vi "_Main_ByRuns_V2.0_3el_5el.vi"() -> ()   [LabVIEW 2017]
uses:
  <vilib>/Instr/_visa.llb/VISA Configure Serial Port (Instr).vi
panel:
  in  "5electrodes":bool=TRUE
  in  "WaveForm":i32(listbox)
  in  "Auto\nturn OFF":bool
  in  "Content":i32(listbox)
  out "LastTrigTimer, s":dbl
  in  "Graph every, cycle":dbl=10.0 min=1.0 max=100.0
  in  "SendPeriod, ms":dbl=100.0 min=10.0 max=10000.0
  out "RunsNeed":i32
  out "DAC1volt, V":dbl
  out "Time LOG":cluster{dbl[], dbl[]}(graph)
  out "LED2":bool
  out "LED1":bool
  out "TrigTimer, s":dbl
  out "Bytes at Port":u32
  out "RecTry":i32
  out "OutVoltage, V":dbl
  out "Field, kV/cm":dbl
  out "VoltageRes, V":dbl
  out "PlotPoints":cluster{"Time":dbl[], "Voltage":dbl[]}(graph)={"Time"=[0.0, 0.00037111111108161925, 0.000510833333311085, 0.0006505555555405509, 0.0007766666666915019, 0.0009172222221968695, 0.0010569444444263353, 0.0011958333333152243, 0.0013350000000274223], "Voltage"=[5.89, 5.89, 5.89, 5.89, 5.89, 5.89, 5.89, 5.89, 5.89]}
  out "VoltageBelow, V":dbl
  in  "Exposition, s":dbl=3.0
  out "Knob":u32
  out "Current, mA":dbl format="%#_4g"
  out "Channel 4, V":dbl format="%#_5g"
  out "Channel 3, V":dbl format="%#_5g"
  out "Channel 2, V":dbl format="%#_5g"
  out "Channel 1, V":dbl format="%#_5g"
  in  "Stop Button":bool
  in  "Start Button":bool
  in  "film H, nm":dbl=50.0
  out "VoltageArray, V":dbl[](array[numeric])
  out "Shutter Red":bool
  out "Shutter Green":bool
  in  "Frames In Run":u32=180
  out "Global Frame Done":u32
  out "Now is Run #":u32
  out "Frame In Run Done":u32
  in  "Step, V":dbl=1.0 min=0.01 max=50.0
  in  "Amplitude, V":dbl=1.0 min=0.1 max=50.0
  in  "LOG file":path
  in  "COM port":refnum<visa-resource-name>
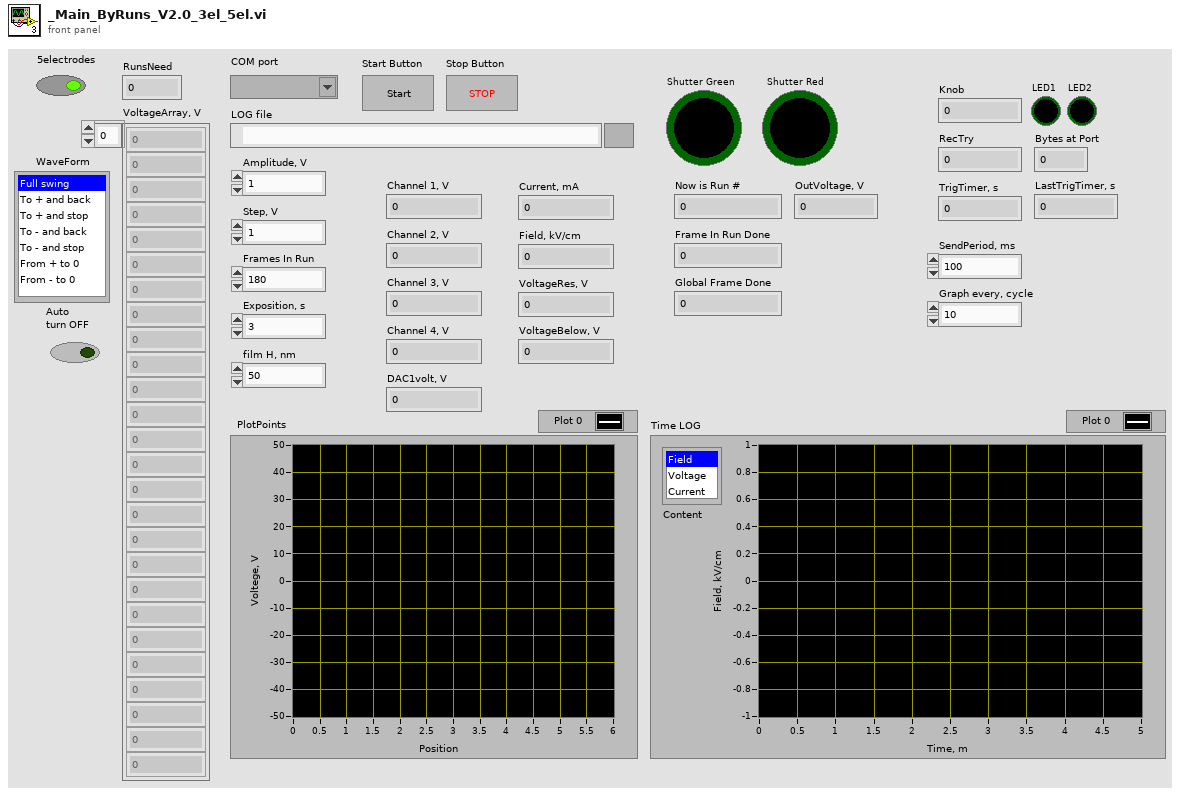
[diagram p1: front panel]
types:
  T1 = cluster{i32, i32, u32, "TrigState":bool, "TrigTimer, s":dbl, "CurrentError":bool}
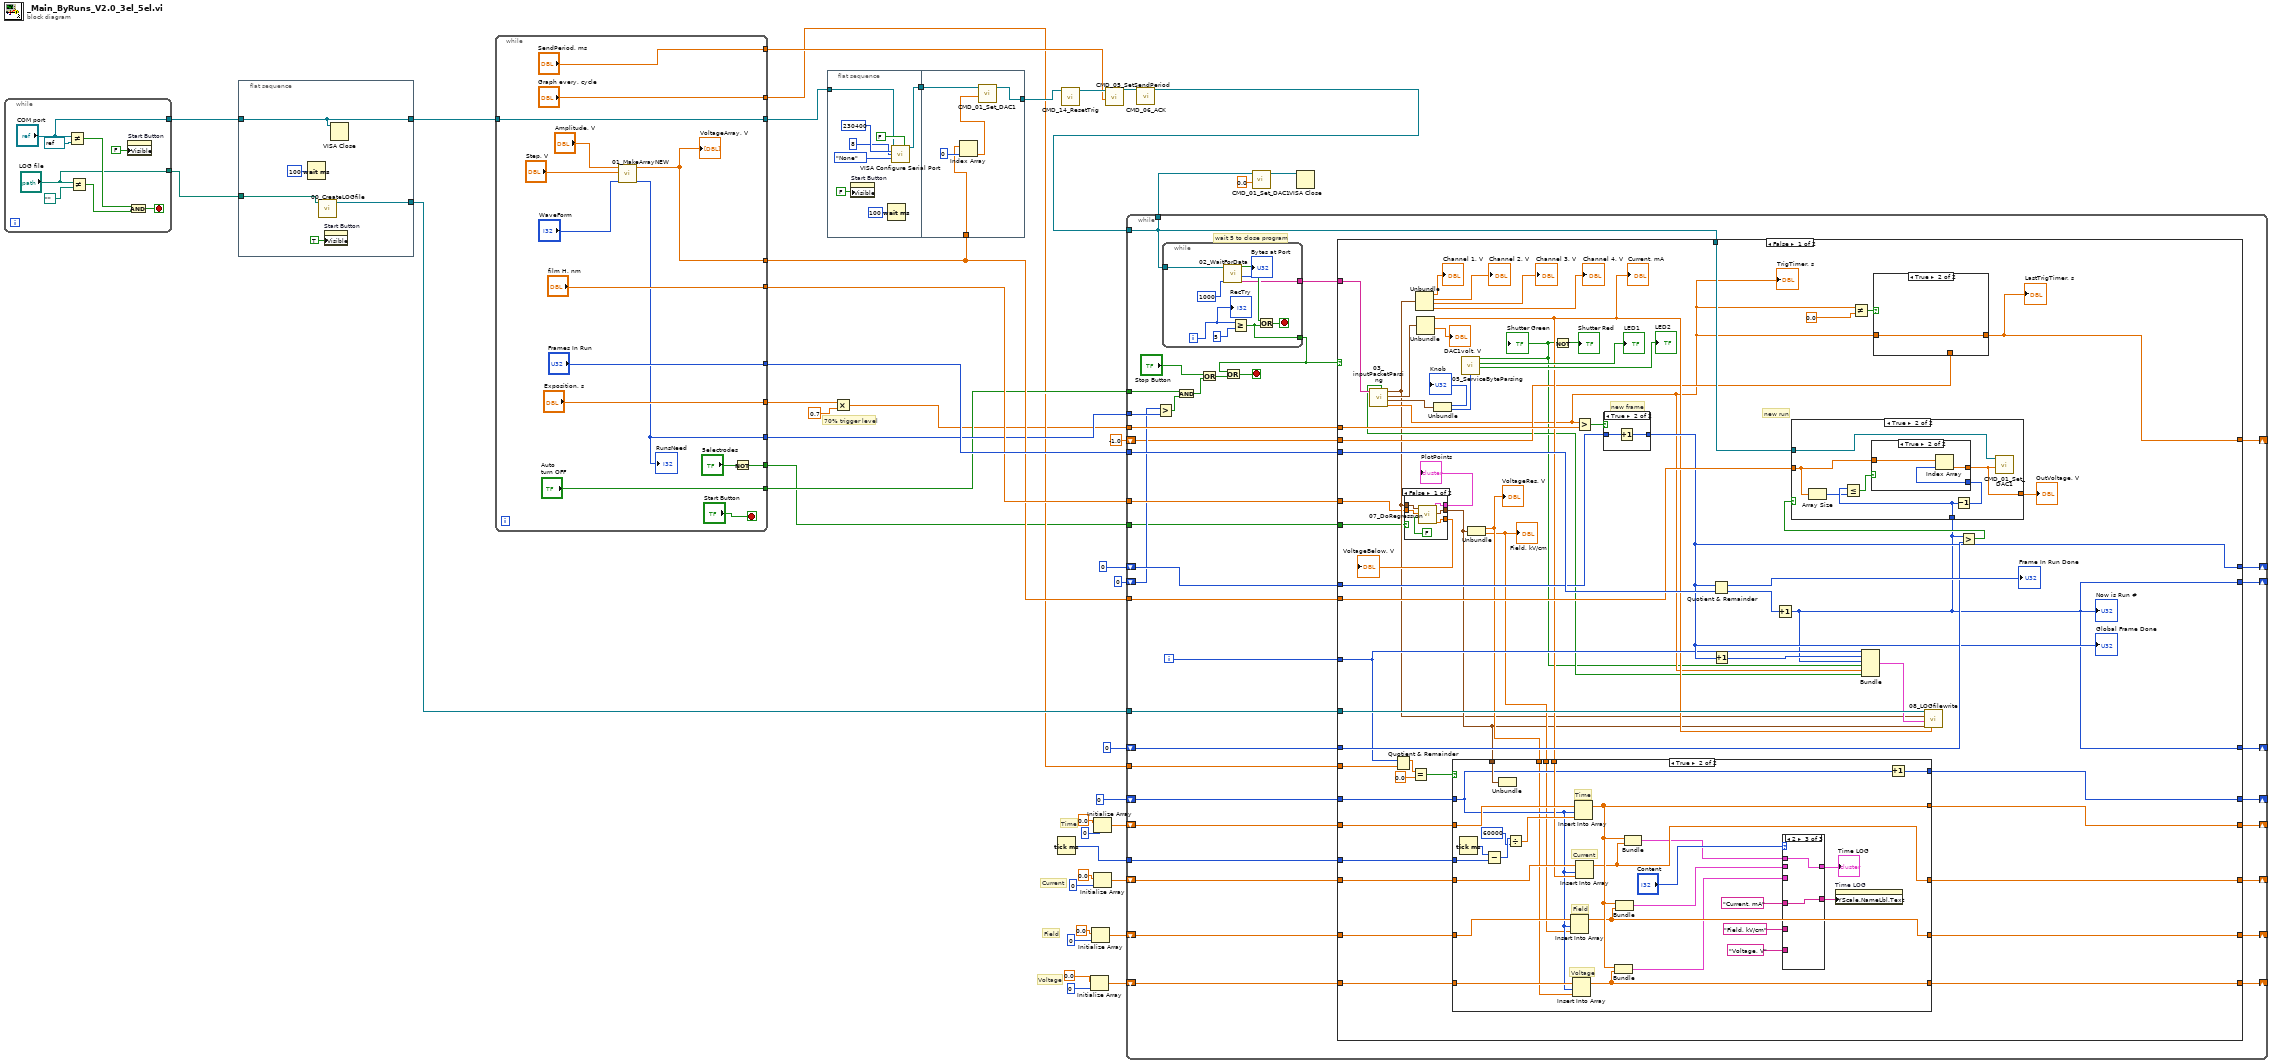
[diagram p0: block diagram]
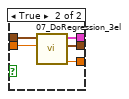
[diagram p2: hidden frame]
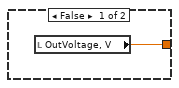
[diagram p7: hidden frame]
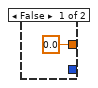
[diagram p8: hidden frame]
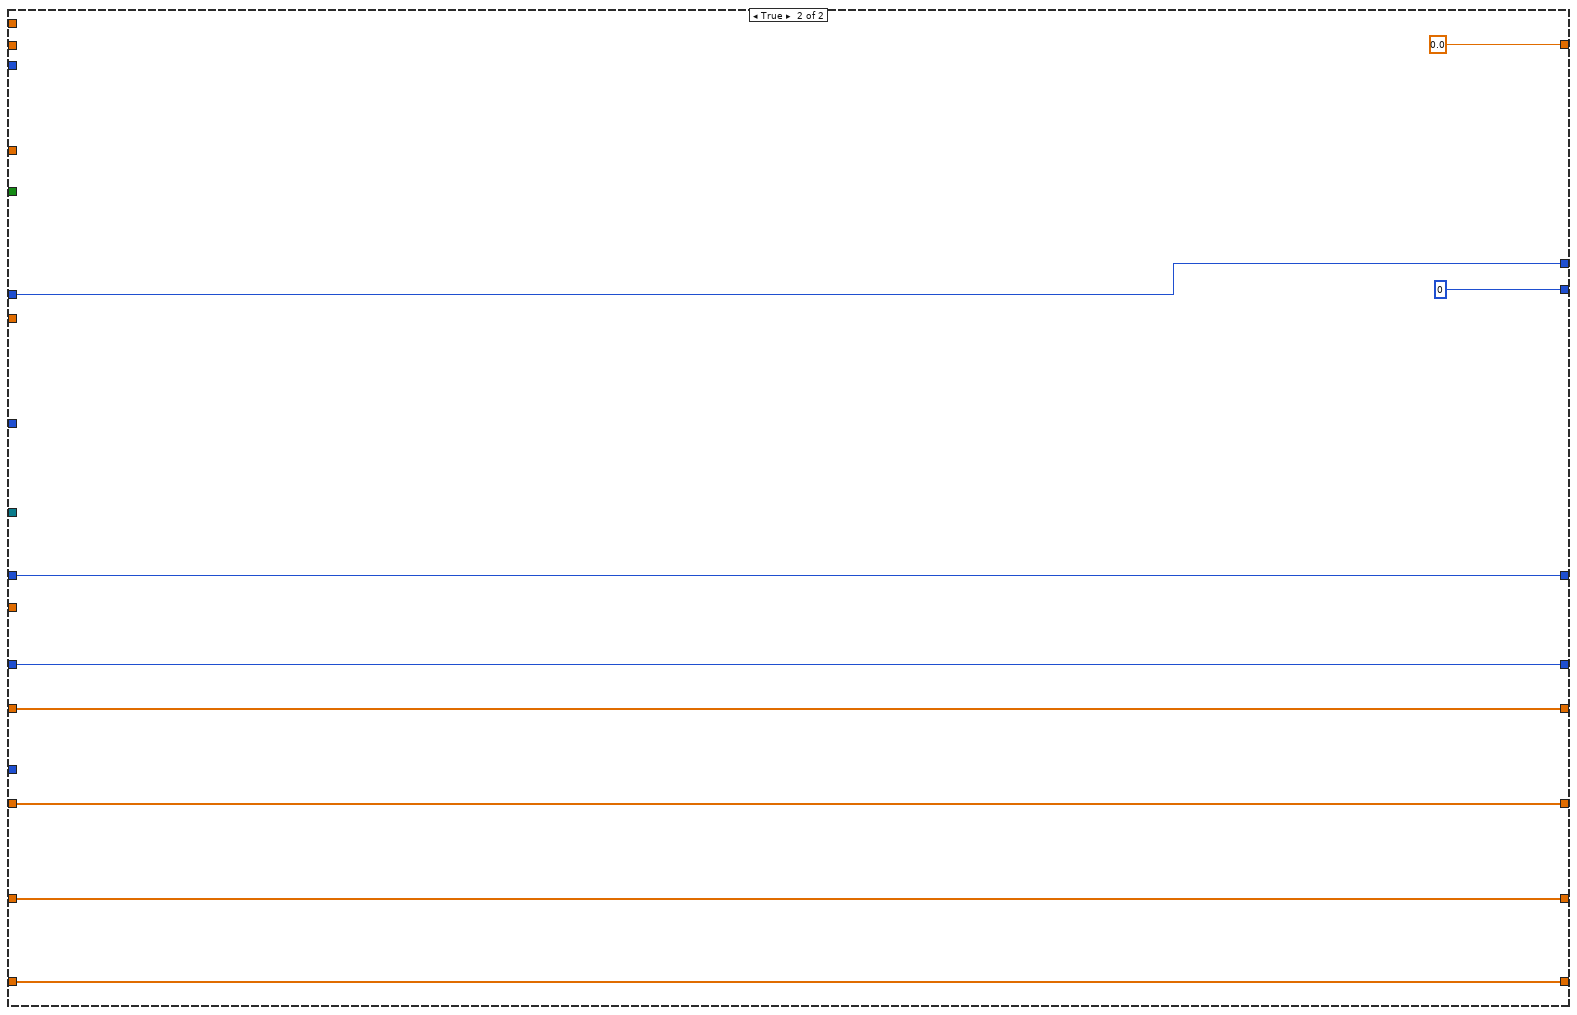
[diagram p10: hidden frame]
diagram:
  # "70% trigger level"
  # "Voltage"
  # "Field"
  # "Time"
  # "Current"
  n1 = while {
    tunnel: ["COM port"] -> w4
    tunnel: ["LOG file"] -> w3
    stop <- w48 stop-if-true
    n2 = Not Equal?(x="COM port", y=refnum<visa-resource-name> refnum ("COM port")) -> (x != y?=w45:bool)
    n3 = Not Equal?(x="LOG file", y=path "" ("LOG file")) -> (x != y?=w46:bool)
    n4 = property on="Start Button" class="Bool"("Visible"=FALSE) -> ()  [unwired: 2 in, 2 out]
    n5 = And(x=w45, y=w46) -> (x .and. y?=w48:bool)
  }
  n6 = flat-sequence {
    tunnel: [w55] -> w39
    tunnel: w4 -> [w51]
    tunnel: w3 -> [w52]
    tunnel: [w51] -> w2
    frame #0 {
      n7 = Wait (ms)(milliseconds to wait=u32 100) -> ()  [unwired: 1 out]
      n8 = call "00_CreateLOGfile.vi"("LOG file"=w52) -> ("refnum out"=w55:refnum<file>)  [unwired: 10 in]
      n9 = property on="Start Button" class="Bool"("Visible"=TRUE) -> ()  [unwired: 2 in, 2 out]
      n10 = VISA Close(VISA resource name=w51) -> ()  [unwired: 1 in, 1 out]
    }
  }
  n11 = while {
    tunnel: w2 -> [w62]
    tunnel: [w62] -> w42
    tunnel: [w59] -> w28
    tunnel: ["film H, nm"] -> w40
    tunnel: ["Frames In Run"] -> w41
    tunnel: ["Exposition, s"] -> w13
    tunnel: [w58] -> w19
    tunnel: ["Auto\nturn OFF"] -> w17
    tunnel: ["SendPeriod, ms"] -> w16
    tunnel: ["Graph every, cycle"] -> w15
    tunnel: [w57] -> w1
    stop <- "Start Button" stop-if-true
    n12 = call "01_MakeArrayNEW.vi"("Amp"="Amplitude, V", "Step"="Step, V", "WaveForm"="WaveForm") -> ("Array"=w59:dbl[], "ArraySize"=w58:i32)  [unwired: 6 in]
    "VoltageArray, V" <- w59
    "RunsNeed" <- w58
    n13 = Not(x="5electrodes") -> (.not. x?=w57:bool)
  }
  n14 = flat-sequence {
    tunnel: w42 -> [w74]
    tunnel: [w73] -> w29
    tunnel: [w81] -> w35
    tunnel: w29 -> [w80]
    tunnel: w28 -> [w79]
    frame #0 {
      n15 = property on="Start Button" class="Bool"("Visible"=FALSE) -> ()  [unwired: 2 in, 2 out]
      n16 = Wait (ms)(milliseconds to wait=u32 100) -> ()  [unwired: 1 out]
      n17 = call-poly "VISA Configure Serial Port"("VISA resource name"=w74, "Enable Termination\nChar (T)"=FALSE ("Enable Termination\nChar (T)"), "baud rate (9600)"=u32 230400, "data bits (8)"=u16 8, "parity (0:none)"=enum16{"None", "Odd", "Even", "Mark", "Space"}."None") -> ("VISA resource name out"=w73:refnum<visa-resource-name>)  [unwired: 9 in, 1 out]
    }
    frame #1 {
      n18 = Index Array(array=w79, index=0) -> (element=w83:dbl)
      n19 = call "CMD_01_Set_DAC1.vi"("Input, V"=w83, "VISA resource name"=w80) -> ("VISA resource name out"=w81:refnum<visa-resource-name>)  [unwired: 9 in]
    }
  }
  n20 = Multiply(x=w13, y=0.7) -> (x*y=w14:dbl)
  n21 = Tick Count (ms)() -> (millisecond timer value=w23:u32)
  n22 = call "CMD_14_ResetTrig.vi"("VISA resource name"=w35) -> ("VISA resource name out"=w32:refnum<visa-resource-name>)  [unwired: 10 in]
  n23 = Initialize Array(0.0 ("element"), 0 ("dimension size")) -> (w5:dbl[])
  n24 = Initialize Array(0.0 ("element"), 0 ("dimension size")) -> (w6:dbl[])
  n25 = Initialize Array(0.0 ("element"), 0 ("dimension size")) -> (w20:dbl[])
  n26 = Initialize Array(0.0 ("element"), 0 ("dimension size")) -> (w24:dbl[])
  n27 = call "CMD_05_SetSendPeriod.vi"("Period, ms"=w16, "VISA resource name"=w32) -> ("VISA resource name out"=w31:refnum<visa-resource-name>)  [unwired: 9 in]
  n28 = call "CMD_06_ACK.vi"("VISA resource name"=w31) -> ("VISA resource name out"=w30:refnum<visa-resource-name>)  [unwired: 10 in]
  n29 = while {
    tunnel: w30 -> [w107]
    tunnel: [w107] -> w36
    tunnel: w28 -> [w108]
    tunnel: w41 -> [w114]
    tunnel: w14 -> [w116]
    tunnel: w40 -> [w117]
    tunnel: w39 -> [w115]
    shift-right: [w111] -> _
    shift-left: 0 -> [w113]
    shift-right: [w110] -> _
    shift-left: u32 0 -> [w109]
    shift-right: [w105] -> _
    shift-left: 0 -> [w106]
    tunnel: w23 -> [w103]
    shift-right: [w101] -> _
    shift-left: w24 -> [w104]
    shift-right: [w100] -> _
    shift-left: w20 -> [w102]
    tunnel: w19 -> [w96]
    shift-right: [w98] -> _
    shift-left: u32 0 -> [w95]
    tunnel: w17 -> [w92]
    tunnel: w15 -> [w91]
    shift-right: [w90] -> _
    shift-left: -1.0 ("TrigTimer, s") -> [w89]
    shift-right: [w86] -> _
    shift-left: w6 -> [w88]
    shift-right: [w85] -> _
    shift-left: w5 -> [w87]
    tunnel: w1 -> [w84]
    i -> [w112]
    stop <- w120 stop-if-true
    # "wait 5 to close program"
    n30 = Greater?(x=w95, y=w96) -> (0:w93:bool)
    n31 = while {
      tunnel: w107 -> [w258]
      tunnel: [w261] -> w119
      tunnel: [w262] -> w118
      i -> [w260]
      stop <- w264 stop-if-true
      n32 = call "02_WaitForData.vi"("WaitTimeoutMS"=u32 1000, "VISA"=w258) -> ("Buffer"=w262:string, "Bytes at Port"=→"Bytes at Port":u32, "Data Recived"=w263:bool)  [unwired: 7 in]
      n33 = Greater Or Equal?(x=w260, y=5) -> (x >= y?=w261:bool)
      n34 = Or(x=w263, y=w261) -> (x .or. y?=w264:bool)
      "RecTry" <- w260
    }
    n35 = And(x=w92, y=w93) -> (x .and. y?=w94:bool)
    n36 = Or(x="Stop Button", y=w94) -> (x .or. y?=w99:bool)
    n37 = Or(x=w119, y=w99) -> (x .or. y?=w120:bool)
    n38 = case shown="False" w119 {
      tunnel: w118 -> [w181 _]
      tunnel: w117 -> [w122 _]
      tunnel: w116 -> [w170 _]
      tunnel: w115 -> [w173 _]
      tunnel: w114 -> [w171 _]
      tunnel: w113 -> [w168 w257]
      tunnel: w112 -> [w152 _]
      tunnel: [w159 w257] -> w111
      tunnel: [w142 w256] -> w110
      tunnel: w109 -> [w162 w256]
      tunnel: w108 -> [w164 _]
      tunnel: w107 -> [w163 _]
      tunnel: w106 -> [w150 w255]
      tunnel: [w149 w255] -> w105
      tunnel: w104 -> [w148 w254]
      tunnel: w103 -> [w147 _]
      tunnel: w102 -> [w146 w253]
      tunnel: [w144 w254] -> w101
      tunnel: [w143 w253] -> w100
      tunnel: [w142 u32 0] -> w98
      tunnel: w91 -> [w140 _]
      tunnel: [w137 0.0 ("TrigTimer, s")] -> w90
      tunnel: w89 -> [w136 _]
      tunnel: w88 -> [w132 w250]
      tunnel: w87 -> [w131 w249]
      tunnel: [w130 w250] -> w86
      tunnel: [w129 w249] -> w85
      tunnel: w84 -> [w121 _]
      frame False {
        # "new run"
        # "new frame"
        n39 = call "03_inputPacketParsing.vi"("string"=w181) -> ("TrigTimer, s"=w135:dbl, "Service state"=w158:cluster{u8, u8}, "DAC state"=w176:cluster{dbl, dbl, dbl, dbl}, "Voltage"=w123:cluster{dbl, dbl, dbl, dbl}, "CurrentError"=w134:bool)  [unwired: 6 in]
        "TrigTimer, s" <- w135
        n40 = Quotient & Remainder(x=w152, y=w140) -> (x-y*floor(x/y)=w154:dbl)  [unwired: 1 out]
        n41 = case shown="False" w121 {
          tunnel: [w182 w192] -> w126
          tunnel: [w183 w191] -> w125
          tunnel: [w184 w190] -> w124
          tunnel: w123 -> [w186 w189]
          tunnel: w122 -> [w185 w188]
          frame False {
            n42 = call "07_DoRegression.vi"("6 electrodes"=FALSE, "film H, nm"=w185, "Input ChVoltage"=w186) -> ("VoltageBelow, V"=w184:dbl, "Regression"=w183:cluster{"VoltageRes, V":dbl, "Field, kV/cm":dbl}, "PlotPoints"=w182:cluster{"Time":dbl[], "Voltage":dbl[]})  [unwired: 6 in]
          }
          frame True {
            n43 = call "07_DoRegression_3el.vi"("film H, nm"=w188, "Input ChVoltage"=w189) -> ("VoltageBelow, V"=w190:dbl, "Regression"=w191:cluster{"VoltageRes, V":dbl, "Field, kV/cm":dbl}, "PlotPoints"=w192:cluster{"Time":dbl[], "Voltage":dbl[]})  [unwired: 7 in]
          }
        }
        "VoltageBelow, V" <- w124
        "PlotPoints" <- w126
        n44 = Equal?(x=w154, y=0.0) -> (x = y?=w151:bool)
        n45 = Unbundle(w123) -> (→"Channel 1, V":dbl, →"Channel 2, V":dbl, →"Channel 3, V":dbl, →"Channel 4, V":dbl)
        n46 = Unbundle(w176) -> (w141:dbl, →"DAC1volt, V":dbl)  [unwired: 2 out]
        "Current, mA" <- w141
        n47 = Unbundle(w158) -> (→"Knob":u8, w157:u8)
        n48 = call "05_ServiceByteParsing.vi"("InputByte"=w157) -> ("LED2"=→"LED2":bool, "LED1"=→"LED1":bool, "TrigState"=w133:bool)  [unwired: 7 in, 1 out]
        "Shutter Green" <- w133
        n49 = Unbundle(w125) -> ("VoltageRes, V"=w128:dbl, "Field, kV/cm"=w127:dbl)
        "VoltageRes, V" <- w128
        "Field, kV/cm" <- w127
        n50 = case shown="True" w151 {
          tunnel: w150 -> [w199 w215]
          tunnel: [w199 w222] -> w149
          tunnel: w125 -> [_ w227]
          tunnel: w148 -> [w197 w220]
          tunnel: w147 -> [_ w225]
          tunnel: w146 -> [w198 w219]
          tunnel: [w198 w209] -> w143
          tunnel: [w197 w212] -> w144
          tunnel: w141 -> [_ w218]
          tunnel: w132 -> [w196 w217]
          tunnel: w131 -> [w195 w216]
          tunnel: [w196 w210] -> w130
          tunnel: [w195 w211] -> w129
          tunnel: w128 -> [_ w213]
          tunnel: w127 -> [_ w214]
          frame False {
          }
          frame True {
            # "Time"
            # "Voltage"
            # "Field"
            # "Current"
            n51 = Tick Count (ms)() -> (millisecond timer value=w226:u32)
            n52 = Subtract(x=w226, y=w225) -> (x-y=w224:u32)
            n53 = Unbundle(w227) -> ()  [unwired: 2 out]
            n54 = Divide(x=w224, y=u32 60000) -> (x/y=w221:dbl)
            n55 = Insert Into Array(array=w217, index=w215, new element=w214) -> (w210:dbl[])
            n56 = Insert Into Array(array=w216, index=w215, new element=w213) -> (w211:dbl[])
            n57 = Insert Into Array(array=w220, index=w215, new element=w221) -> (w212:dbl[])
            n58 = Insert Into Array(array=w219, index=w215, new element=w218) -> (w209:dbl[])
            n59 = Bundle(w212, w211) -> (w205:cluster{dbl[], dbl[]})  [unwired: 1 in]
            n60 = Bundle(w212, w210) -> (w206:cluster{dbl[], dbl[]})  [unwired: 1 in]
            n61 = Bundle(w212, w209) -> (w207:cluster{dbl[], dbl[]})  [unwired: 1 in]
            n62 = case shown="2" "Content" {
              tunnel: w207 -> [_ _ w233]
              tunnel: w206 -> [w229 _ _]
              tunnel: w205 -> [_ w231 _]
              tunnel: [w229 w231 w233] -> w204
              tunnel: "Current, mA" ("Y Scale.Name Label.Text") -> [_ _ w232]
              tunnel: "Field, kV/cm" ("Y Scale.Name Label.Text") -> [w228 _ _]
              tunnel: "Voltage, V" ("Y Scale.Name Label.Text") -> [_ w230 _]
              tunnel: [w228 w230 w232] -> w200
              frame 0, Default {
              }
              frame 1 {
              }
              frame 2 {
              }
            }
            "Time LOG" <- w204
            n63 = property on="Time LOG" class="XYGraph (strict)"("YScale.NameLbl.Text"=w200) -> ()  [unwired: 2 in, 2 out]
            n64 = Increment(x=w215) -> (x+1=w222:i32)
          }
        }
        n65 = Not(x=w133) -> (.not. x?=→"Shutter Red":bool)
        n66 = Greater?(x=w135, y=w170) -> (0:w169:bool)
        n67 = case shown="True" w169 {
          tunnel: w168 -> [w246 w248]
          tunnel: [w246 w247] -> w159
          frame False {
          }
          frame True {
            n68 = Increment(x=w248) -> (x+1=w247:i32)
          }
        }
        "Global Frame Done" <- w159
        n69 = Quotient & Remainder(x=w159, y=w171) -> (x-y*floor(x/y)=→"Frame In Run Done":u32, floor(x/y)=w166:u32)
        n70 = Increment(x=w159) -> (x+1=w160:i32)
        n71 = Increment(x=w166) -> (x+1=w142:u32)
        "Now is Run #" <- w142
        n72 = Not Equal?(x=w135, y=0.0) -> (x != y?=w139:bool)
        n73 = Bundle(w152, w160, w142, "TrigState"=w133, "TrigTimer, s"=w135, "CurrentError"=w134) -> (w172:T1)  [unwired: 1 in]
        n74 = case shown="True" w139 {
          tunnel: [w193 w194] -> w137
          tunnel: w135 -> [_ w194]
          tunnel: w136 -> [w193 _]
          frame False {
          }
          frame True {
          }
        }
        "LastTrigTimer, s" <- w137
        n75 = call "08_LOGfilewrite.vi"("DAC1cur"=w141, "Regression"=w125, "Counters"=w172, "Input ChVoltage"=w123, "refnum out"=w173) -> ()  [unwired: 7 in]
        n76 = Greater?(x=w142, y=w162) -> (0:w167:bool)
        n77 = case shown="True" w167 {
          tunnel: w164 -> [_ w237]
          tunnel: w142 -> [_ w240]
          tunnel: w163 -> [_ w236]
          tunnel: [w234 w235] -> w161
          frame False {
            n78 = local read "OutVoltage, V"() -> (w234:dbl)
          }
          frame True {
            n79 = Array Size(array=w237) -> (size(s)=w239:i32)
            n80 = Less Or Equal?(x=w240, y=w239) -> (x <= y?=w238:bool)
            n81 = Decrement(x=w240) -> (x-1=w241:u32)
            n82 = case shown="True" w238 {
              tunnel: w241 -> [_ w245]
              tunnel: w237 -> [_ w244]
              tunnel: [0.0 w243] -> w235
              frame False {
              }
              frame True {
                n83 = Index Array(array=w244, index=w245) -> (element=w243:dbl)
              }
            }
            n84 = call "CMD_01_Set_DAC1.vi"("Input, V"=w235, "VISA resource name"=w236) -> ()  [unwired: 9 in, 1 out]
          }
        }
        "OutVoltage, V" <- w161
      }
      frame True {
      }
    }
  }
  n85 = call "CMD_01_Set_DAC1.vi"("Input, V"=0.0, "VISA resource name"=w36) -> ("VISA resource name out"=w33:refnum<visa-resource-name>)  [unwired: 9 in]
  n86 = VISA Close(VISA resource name=w33) -> ()  [unwired: 1 in, 1 out]
